vi "change channel settings.vi"(6 "channel classification":T1, 8 "error in":errorcluster, 9 "data type":T2, 10 "channel name":string, 11 "Scan Engine editor node in":refnum<class "Scan Engine editor node.lvclass">) -> (0 "error out":errorcluster, 3 "Scan Engine editor node out":refnum<class "Scan Engine editor node.lvclass">)   [LabVIEW 2013, in "Scan Engine editor node.lvclass"]
uses:
  Scan Engine editor node.lvclass
  <vilib>/NI/Tag Bus/tag/Data Type.ctl
  <vilib>/NI/Tag Bus Module Framework/channel/channel classification.ctl
  <vilib>/NI/TBM Modules/variable/module/configuration/Scan Engine configuration.lvclass
  <vilib>/NI/Tag Bus/tag/tag descriptor.lvclass/tag descriptor.ctl
  <vilib>/NI/Tag Bus Module Framework/channel/TBM channel.lvclass/TBM channel.ctl
  <vilib>/NI/Tag Bus/tag/read tag name.vi
  read actual configuration.vi
  write actual configuration.vi
  <vilib>/NI/Tag Bus Module Framework/channel/TBM channel.lvclass
  <vilib>/NI/Tag Bus/tag/tag descriptor.lvclass
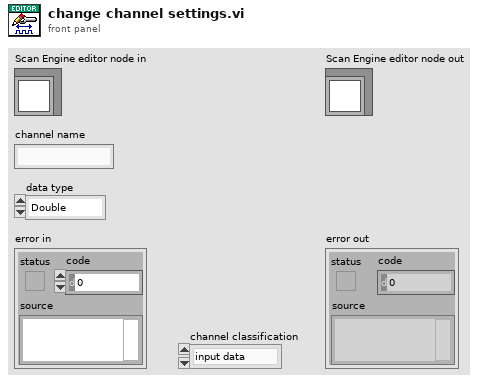
[diagram p1: front panel]
types:
  T1 = typedef "TBM channel.lvclass/channel classification.ctl" = enum16{"input data", "output data", "processing parameter", "processing result"}
  T2 = typedef "tag bus.lvlib/tag descriptor.lvclass/Data Type.ctl" = enum16{"Double", "Single", "I64", "I32", "I16", "I8", "U64", "U32", "U16", "U8", "Boolean", "String", "Array of Double", "Array of Single", "Array of I64", "Array of I32", "Array of I16", "Array of I8", "Array of U64", "Array of U32", "Array of U16", "Array of U8", "Array of Boolean", "Array of String"}
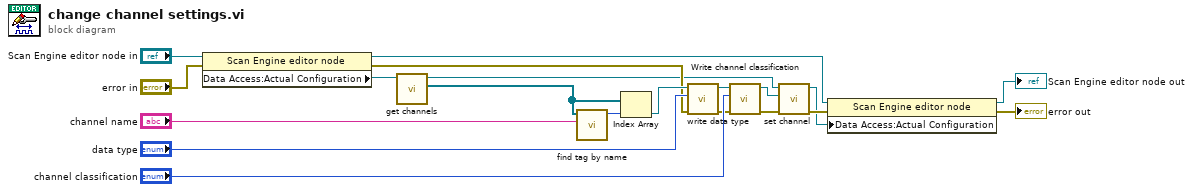
[diagram p0: block diagram]
diagram:
  n1 = property class="Scan Engine editor node"(reference="Scan Engine editor node in", error in="error in") -> (reference out=w17:refnum<class "Scan Engine editor node.lvclass">, error out=w4:errorcluster, "Data Access:Actual Configuration"=w2:refnum<class "Scan Engine configuration.lvclass">)
  n2 = call-dynamic "get channels.vi"("module configuration in"=w2) -> ("channels"=w3:refnum<class "TBM channel.lvclass">[], "module configuration out"=w1:refnum<class "Scan Engine configuration.lvclass">)  [unwired: 9 in]
  n3 = call <vilib>:"find tag by name.vi"("name"="channel name", "tags in"=w3) -> ("index"=w7:i32)  [unwired: 9 in]
  n4 = Index Array(array=w3, index=w7) -> (element=w6:refnum<class "TBM channel.lvclass">)
  n5 = call <vilib>:"write data type.vi"("error in"=w4, "data type"="data type", "system tag in"=w6) -> ("error out"=w11:errorcluster, "system tag out"=w15:refnum<class "TBM channel.lvclass">)  [unwired: 7 in]
  n6 = call <vilib>:"Write channel classification.vi"("error in"=w11, "channel classification"="channel classification", "channel in"=w15) -> ("error out"=w12:errorcluster, "channel out"=w5:refnum<class "TBM channel.lvclass">)  [unwired: 7 in]
  n7 = call <vilib>:"set channel.vi"("error in"=w12, "channel"=w5, "Scan Engine configuration in"=w1) -> ("error out"=w10:errorcluster, "Scan Engine configuration out"=w9:refnum<class "Scan Engine configuration.lvclass">)  [unwired: 7 in]
  n8 = property class="Scan Engine editor node"(reference=w17, error in=w10, "Data Access:Actual Configuration"=w9) -> (reference out=→"Scan Engine editor node out":refnum<class "Scan Engine editor node.lvclass">, error out=→"error out":errorcluster)
